vi "GDSProject_OpenClass.vi"(1 "ClassPath(FilePath/ProjectTreePath/LvCLassRef)":variant, 5 "error IO":errorcluster) -> (15 "LVClass.Open":refnum<vi>, 16 "LvClassCreated":bool, 19 "error out":errorcluster)   [LabVIEW 2014]
uses:
  <resource>/Framework/Providers/Open_GDS/ClassProviders/Provider_EndevoGOOP300/ClassWriterGOOP300_class/ClassWriterGOOP300.lvclass
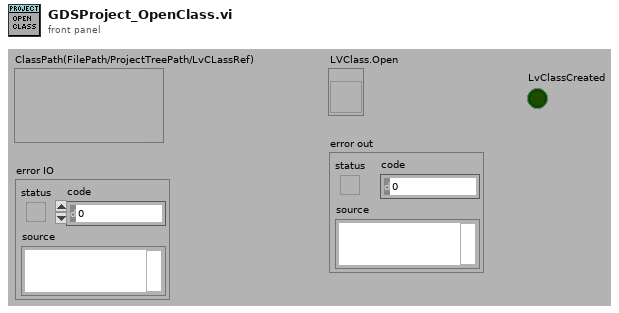
[diagram p1: front panel]
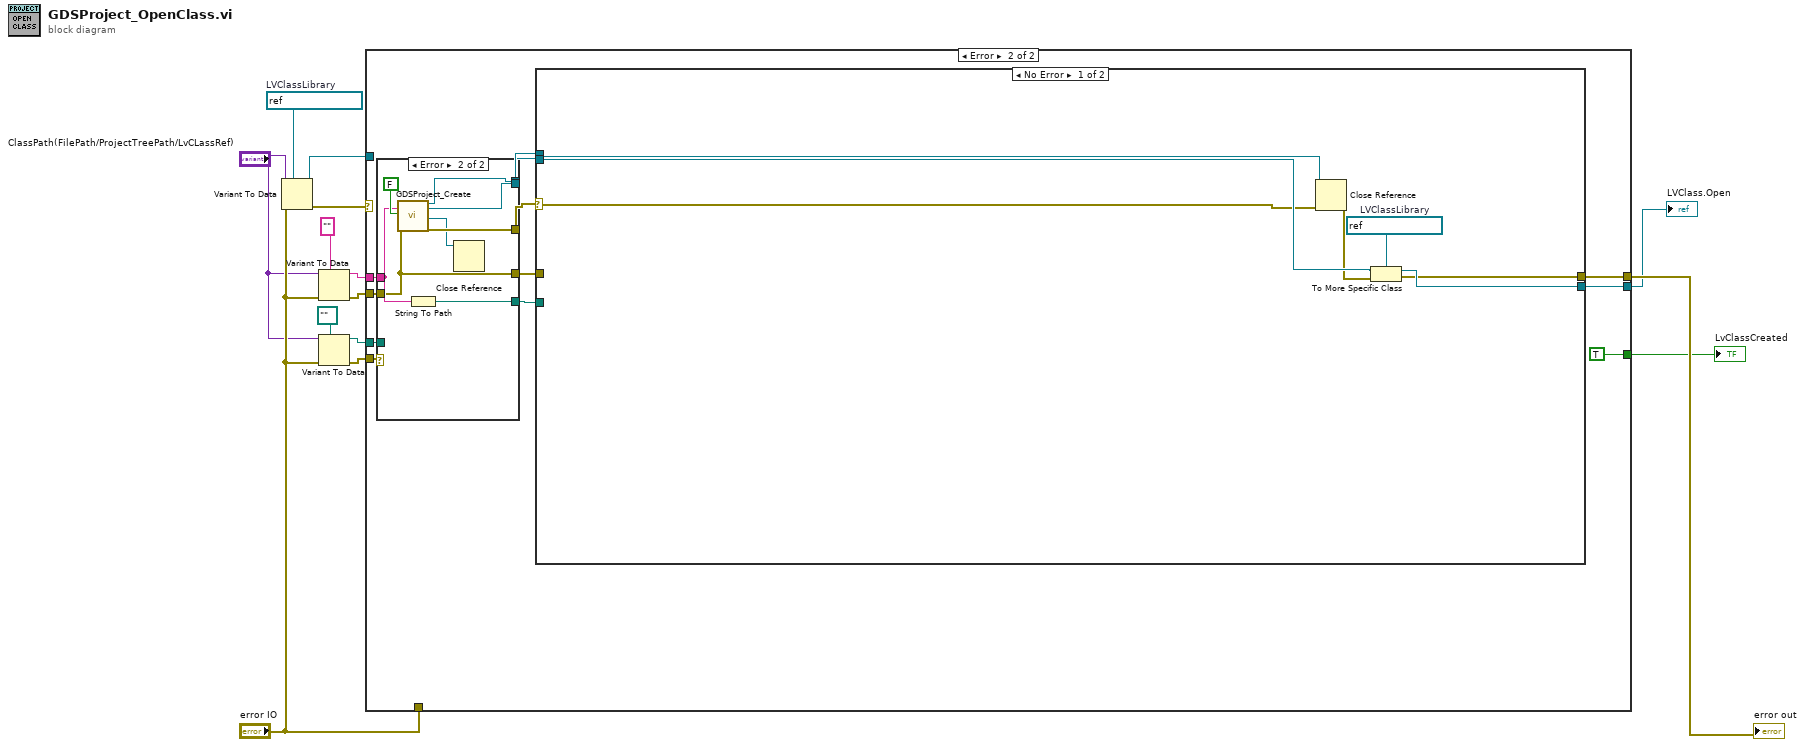
[diagram p0: block diagram]
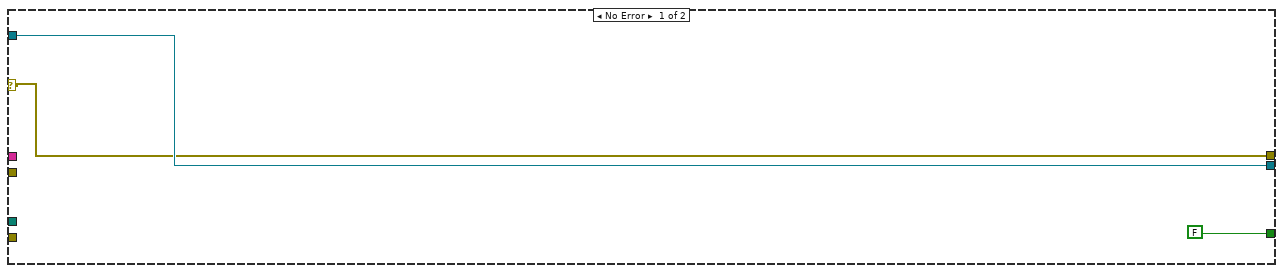
[diagram p2: hidden frame]
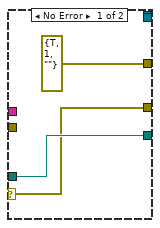
[diagram p3: hidden frame]
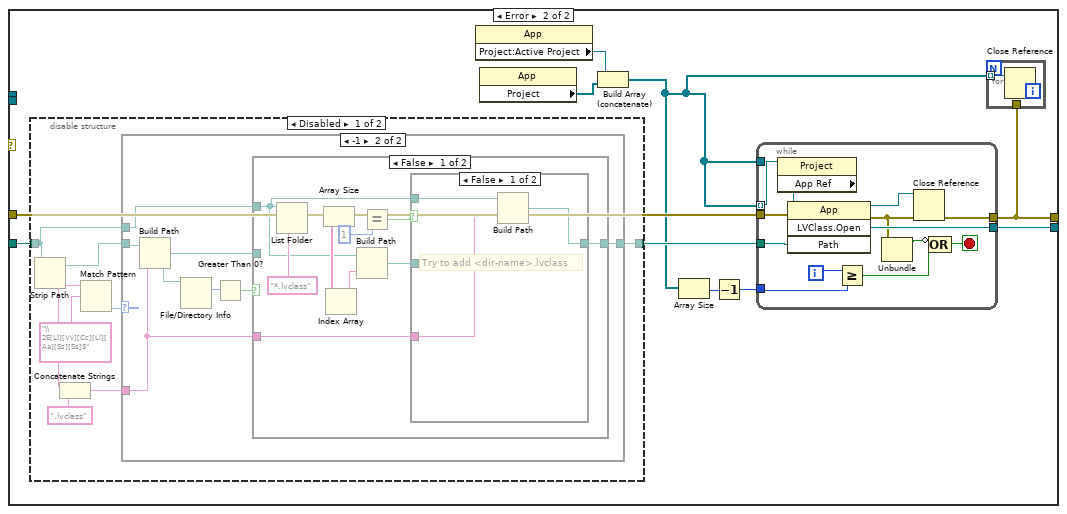
[diagram p4: hidden frame]
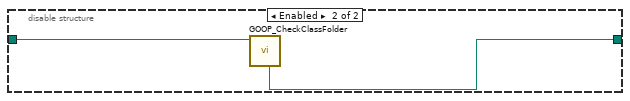
[diagram p8: hidden frame]
diagram:
  w9 = refnum<vi> refnum  # LVClassLibrary
  n1 = Variant To Data(error in="error IO", type=w9, Variant="ClassPath(FilePath/ProjectTreePath/LvCLassRef)") -> (data=w11:refnum<vi>, error out=w10:errorcluster)
  n2 = Variant To Data(error in="error IO", type="", Variant="ClassPath(FilePath/ProjectTreePath/LvCLassRef)") -> (data=w14:string, error out=w13:errorcluster)
  n3 = Variant To Data(error in="error IO", type=path "", Variant="ClassPath(FilePath/ProjectTreePath/LvCLassRef)") -> (data=w2:path, error out=w3:errorcluster)
  n4 = case shown="Error" w10 {
    selector: w10 -> [w16 _]
    tunnel: [w17 w26] -> w7
    tunnel: "error IO" -> [_ _]
    tunnel: [w16 w25] -> w8
    tunnel: w11 -> [w17 _]
    tunnel: w13 -> [_ w23]
    tunnel: w14 -> [_ w22]
    tunnel: w3 -> [_ w21]
    tunnel: w2 -> [_ w20]
    tunnel: [FALSE TRUE] -> w1
    frame No Error {
    }
    frame Error {
      n5 = case shown="Error" w21 {
        selector: w21 -> [w30 _]
        tunnel: [_ w40] -> w29
        tunnel: [errorcluster {"status"=TRUE, "code"=1, "source"=""} ("error out") w38] -> w28
        tunnel: [w31 w37] -> w27
        tunnel: [_ w36] -> w24
        tunnel: w23 -> [_ w34]
        tunnel: w22 -> [_ w35]
        tunnel: w20 -> [w31 _]
        tunnel: [w30 w34] -> w19
        frame No Error {
        }
        frame Error {
          n6 = call <resource>:"GDSProject_Create.vi"("ProjectTreePosition(String or Project Item Ref)"=w35, "AllowPopUpDilaog(True)"=FALSE, "error in (no error)"=w34) -> ("Project Refnum"=w40:refnum<vi>, "Project Item"=w36:refnum<vi>, "App"=w33:refnum<vi>, "error out"=w38:errorcluster)  [unwired: 13 in]
          n7 = String To Path(string=w35) -> (path=w37:path)
          n8 = Close Reference(reference=w33) -> ()  [unwired: 1 in, 1 out]
        }
      }
      n9 = case shown="No Error" w28 {
        selector: w28 -> [w42 _]
        tunnel: w29 -> [w47 _]
        tunnel: w27 -> [_ w52]
        tunnel: [w44 w57] -> w26
        tunnel: [w43 w51] -> w25
        tunnel: w19 -> [_ w56]
        tunnel: w24 -> [w46 _]
        frame No Error {
          w45 = refnum<vi> refnum  # LVClassLibrary
          n10 = Close Reference(reference=w47, error in (no error)=w42) -> (error out=w41:errorcluster)
          n11 = To More Specific Class(target class=w45, reference=w46, error in=w41) -> (specific class reference=w44:refnum<vi>, error out=w43:errorcluster)
        }
        frame Error {
          n12 = disable-structure shown="Disabled" {
            disable-tunnel: [w63 w89] -> w53
            disable-tunnel: w52 -> [w58 w90]
            frame Disabled {
              n13 = Strip Path(path=w58) -> (stripped path=w59:path, name=w62:string)
              n14 = Concatenate Strings(w62, ".lvclass" ("string")) -> (w60:string)
              n15 = Match Pattern(string=w62, regular expression="\\2E[Ll][Vv][Cc][Ll][Aa][Ss][Ss]$") -> (offset past match=w64:i32)  [unwired: 1 in, 3 out]
              n16 = case shown="-1" w64 {
                tunnel: w59 -> [_ w68]
                tunnel: [w66 w70] -> w63
                tunnel: w60 -> [_ w67]
                tunnel: w58 -> [w66 w69]
                frame 0, Default {
                  # "It's a lvclassFile"
                }
                frame -1 {
                  n17 = Build Path(base path=w68, name or relative path=w67) -> (appended path=w71:path)
                  n18 = File/Directory Info(path=w71) -> (size=w73:i64)  [unwired: 1 in, 6 out]
                  n19 = Greater Than 0?(x=w73) -> (x > 0?=w72:bool)
                  n20 = case shown="False" w72 {
                    tunnel: w71 -> [_ w88]
                    tunnel: [w77 w88] -> w70
                    tunnel: w69 -> [w75 _]
                    tunnel: w67 -> [w74 _]
                    frame False {
                      n21 = List Folder(path=w75, pattern="*.lvclass" ("string")) -> (filenames=w80:string[])  [unwired: 2 in, 3 out]
                      n22 = Array Size(array=w80) -> (size(s)=w82:i32)
                      n23 = Index Array(array=w80) -> (element=w79:string)  [unwired: 1 in]
                      n24 = Build Path(base path=w75, name or relative path=w79) -> (appended path=w76:path)
                      n25 = Equal?(x=w82, y=1) -> (x = y?=w78:bool)
                      n26 = case shown="False" w78 {
                        tunnel: [w85 w87] -> w77
                        tunnel: w76 -> [_ w87]
                        tunnel: w75 -> [w86 _]
                        tunnel: w74 -> [w84 _]
                        frame False {
                          # "Try to add <dir-name>.lvclass"
                          n27 = Build Path(base path=w86, name or relative path=w84) -> (appended path=w85:path)
                        }
                        frame True {
                          # "Just needed to search for\nlvclass files in this dir"
                        }
                      }
                    }
                    frame True {
                      # "Just needed to Add .lvclass"
                    }
                  }
                }
              }
            }
            frame Enabled {
              n28 = call <resource>:"GOOP_CheckClassFolder.vi"("Class Or Class Floder"=w90) -> ("ClassPath"=w89:path)  [unwired: 6 in, 4 out]
            }
          }
          n29 = property class="App"() -> ("Project:Active Project"=w50:refnum<vi>)  [unwired: 2 in, 2 out]
          n30 = property class="App"() -> ("Project"=w49:refnum<vi>[])  [unwired: 2 in, 2 out]
          n31 = Build Array (concatenate)(w50, w49) -> (w48:refnum<vi>[])
          n32 = Array Size(array=w48) -> (size(s)=w55:i32)
          n33 = Decrement(x=w55) -> (x-1=w54:i32)
          n34 = while {
            tunnel: w53 -> [w104]
            tunnel: [w103] -> w57
            tunnel: w56 -> [w102]
            tunnel: w48 -> [w96] mode=indexing
            tunnel: w54 -> [w100]
            tunnel: w48 -> [_]
            tunnel: [w92] -> w51
            i -> [w101]
            stop <- w97 stop-if-true
            n35 = property class="Project"(reference=w96) -> ("App Ref"=w95:refnum<vi>)  [unwired: 1 in, 2 out]
            n36 = invoke class="App" method="LVClass.Open"(reference=w95, error in=w102, "Path"=w104) -> (reference out=w93:refnum<vi>, error out=w94:errorcluster, "LVClass.Open"=w103:refnum<vi>)  [unwired: 1 in, 1 out]
            n37 = Greater Or Equal?(x=w101, y=w100) -> (x >= y?=w98:bool)
            n38 = Unbundle(w94) -> ("status"=w99:bool)  [unwired: 2 out]
            n39 = Close Reference(reference=w93, error in (no error)=w94) -> (error out=w92:errorcluster)
            n40 = Compound Arithmetic op=OR(invert w99, w98) -> (w97:bool)
          }
          n41 = for {
            tunnel: w48 -> [w91] mode=indexing
            tunnel: w51 -> [_]
            n42 = Close Reference(reference=w91) -> ()  [unwired: 1 in, 1 out]
          }
        }
      }
    }
  }
  "error out" <- w8
  "LVClass.Open" <- w7
  "LvClassCreated" <- w1
